vi "Main Tclk.vi"() -> ()   [LabVIEW 2018] (continued)
                        n6809 = Build Path(base path=w1551, name or relative path=w1554) -> (appended path=w1552:path)
                        n6810 = File/Directory Info(path=w1552) -> (path out=w1557:path, error out=w1555:errorcluster)  [unwired: 1 in, 5 out]
                        n6811 = Unbundle By Name(w1555) -> ("status"=w1556:bool)
                        n6812 = case shown="True" w1556 {
                          tunnel: w1557 -> [_ w1571]
                          frame False {
                          }
                          frame True {
                            n6813 = Create Folder(path (use dialog)=w1571) -> ()  [unwired: 1 in, 4 out]
                          }
                        }
                      }
                      frame #1 {
                        n6814 = call "Read FIB Log Files.vi"("Log file path"=path "C:/Program Files (x86)/FEI Company/BDS/LogHVData.log") -> ("HV Data Output"=w1578:T113)  [unwired: 9 in, 1 out]
                        n6815 = Unbundle By Name(w1578) -> ("Filament (A)"=w1594:sgl, "Acclerator (V)"=w1593:sgl, "AccI (uA)"=w1592:sgl, "Extractor (V)"=w1591:sgl, "Emission (uA)"=w1579:sgl, "Suppressor (V)"=w1580:sgl, "SuppI (uA)"=w1590:sgl, "Lens1 (V)"=w1589:sgl, "Lens1I (uA)"=w1588:sgl, "Lens2 (V)"=w1587:sgl, "Lens2I (uA)"=w1586:sgl, "Tip Lifetime (hr)"=w1577:sgl)
                        n6816 = local read "Faraday Cup RT"() -> (w1575:sgl)
                        n6817 = local read "Specimen RT"() -> (w1574:sgl)
                        n6818 = local read "BD1 RT"() -> (w1573:sgl)
                        n6819 = local read "BD2 RT"() -> (w1572:sgl)
                        n6820 = Build Array(w1594, w1593, w1592, w1591, w1579, w1580, w1590, w1589, w1588, w1587, w1586, w1577, w1575, w1574, w1573, w1572) -> (w1582:sgl[])
                        n6821 = Bundle("Suppressor (V)"=w1580, "Emission (uA)"=w1579) -> (w1581:T117)  [unwired: 1 in]
                        n6822 = Add Array Elements(numeric array=w1582) -> (sum=w1583:sgl)
                        n6823 = Equal To 0?(x=w1583) -> (x = 0?=w1585:bool)
                        n6824 = Equal To 0?(x=w1577) -> (x = 0?=w1584:bool)
                        n6825 = And(x=w1585, y=w1584) -> (x .and. y?=w1576:bool)
                        "Re-read HVDataLog" <- w1576
                        n6826 = case shown="False" w1576 {
                          tunnel: w1582 -> [w1599 _]
                          tunnel: w1581 -> [w1603 _]
                          tunnel: w1578 -> [w1596 _]
                          frame False {
                            n6827 = local read "FIB HV DataLog Files"() -> (w1601:path)
                            n6828 = Get Date/Time In Seconds() -> (seconds since 1Jan1904=w1600:timestamp)
                            n6829 = for {
                              tunnel: w1599 -> [w1605] mode=indexing
                              tunnel: [w1604] -> w1598 mode=indexing
                              n6830 = Format Into String(w1605) -> (resulting string=w1604:string)  [unwired: 3 in, 1 out]
                            }
                            n6831 = call "YMD log files.vi"("Input text array"=w1598, "Input header array"=string[] ["Date", "Time", "Filament Current (A)", "Accelerator (V)", "Accelerator I (uA)", "Extractor (V)", "Emission (uA)", "Suppressor (V)", "Suppressor I (uA)", "Lens 1 (V)", "Lens 1 I (uA)", "Lens 2 (V)", "Lens 2 I (uA)", "Tip Lifetime (hr)", "Faraday Cup (nA)", "Specimen (nA)", "Beam Dump 1 (nA)", "Beam Dump 2 (nA)"], "current time"=w1600, "Log file name"="HVDataLog" ("string"), "Log file path"=w1601) -> ()  [unwired: 7 in]
                            "FIB HV DataLog" <- w1603
                            "HV Data Output" <- w1596
                          }
                          frame True {
                          }
                        }
                      }
                    }
                  }
                }
                n6832 = Add(x=w1544, y=w1543) -> (x+y=w1547:u32)
                n6833 = expression code="x*1000"("Interval (s)") -> (w1542:u16)
                n6834 = Less?(x=w1547, y=w1542) -> (x < y?=w1548:bool)
                n6835 = Select(t=w1547, s=w1548, f=u32 0) -> (s? t:f=w1545:u32)
                n6836 = property on="FIB HV DataLog" class="WFChart (strict)"("XScale.Multiplier"="Interval (s)") -> ()  [unwired: 2 in, 2 out]
              }
              frame 1, Default {
              }
              frame 2 {
                n6837 = Equal To 0?(x=w1611) -> (x = 0?=w1614:bool)
                n6838 = local read "Re-read HVDataLog"() -> (w1615:bool)
                n6839 = Or(x=w1614, y=w1615) -> (x .or. y?=w1608:bool)
                n6840 = case shown="True" w1608 {
                  tunnel: w1607 -> [_ w1619]
                  frame False {
                  }
                  frame True {
                    n6841 = stacked-sequence {
                      tunnel: w1619 -> [w1623 _]
                      frame #0 {
                        n6842 = local read "FIB HV DataLog Files"() -> (w1624:path)
                        n6843 = local read "Api"() -> (w1620:refnum<k7>)
                        n6844 = call "SmartSEM Remote API get FIB HV data.vi"("Api in"=w1620) -> ("error out"=w1622:errorcluster, "Capella HV Data Output"=w1621:T17)  [unwired: 7 in, 2 out]
                        n6845 = Get Date/Time In Seconds() -> (seconds since 1Jan1904=w1631:timestamp)
                        n6846 = local write "Capella HV Data Output"(w1621) -> ()
                        n6847 = Format Date/Time String(time format string (%c)="Y%Y\\M%m\\D%d", seconds (now)=w1631) -> (date/time string=w1627:string)  [unwired: 1 out]
                        n6848 = Build Path(base path=w1624, name or relative path=w1627) -> (appended path=w1625:path)
                        n6849 = File/Directory Info(path=w1625) -> (path out=w1630:path, error out=w1628:errorcluster)  [unwired: 1 in, 5 out]
                        n6850 = case shown="True" w1623 {
                          tunnel: w1622 -> [_ _]
                          frame False {
                          }
                          frame True {
                            w1633 = 0.0
                            n6851 = Get Date/Time In Seconds() -> (seconds since 1Jan1904=w1643:timestamp)
                            n6852 = To Double Precision Float(number=w1643) -> (double precision float=w1638:dbl)
                            n6853 = Bundle(w1633, w1633) -> (w1632:cluster{dbl, dbl})  [unwired: 1 in]
                            n6854 = Add(x=w1638, y=86400.0 ("X Scale.Range:Maximum")) -> (x+y=w1640:dbl)
                            n6855 = Initialize Array(w1632, 0) -> (w1635:cluster{dbl, dbl}[])
                            n6856 = Add(x=w1638, y=0.0 ("X Scale.Range:Minimum")) -> (x+y=w1636:dbl)
                            n6857 = property on="FIB HV DataLog" class="WFChart (strict)"("History Data"=w1635, "XScale.Offset"=w1638, "XScale.Minimum"=w1636, "XScale.Maximum"=w1640, "XScale.Increment"=14400.0 ("X Scale.Range:Increment"), "XScale.MinorInc"=3600.0 ("X Scale.Range:Minor Increment")) -> ()  [unwired: 2 in, 2 out]
                          }
                        }
                        n6858 = Unbundle By Name(w1628) -> ("status"=w1629:bool)
                        n6859 = case shown="True" w1629 {
                          tunnel: w1630 -> [_ w1644]
                          frame False {
                          }
                          frame True {
                            n6860 = Create Folder(path (use dialog)=w1644) -> ()  [unwired: 1 in, 4 out]
                          }
                        }
                      }
                      frame #1 {
                        n6861 = local read "Capella HV Data Output"() -> (w1645:T17)
                        n6862 = Unbundle By Name(w1645) -> ("Filament (A)"=w1666:sgl, "Accelerator Target (V)"=w1665:sgl, "Accelerator Actual (V)"=w1664:sgl, "Extrator Target (V)"=w1663:sgl, "Extrator Actual (V)"=w1662:sgl, "Emission Target (uA)"=w1661:sgl, "Emission Actual (uA)"=w1654:sgl, "Suppressor (V)"=w1655:sgl, "Lens1 Target (V)"=w1660:sgl, "Lens1 Actual (V)"=w1659:sgl, "Lens2 Target (V)"=w1658:sgl, "Lens2 Actual (V)"=w1657:sgl, "Tip Lifetime (uAhr)"=w1653:sgl, "Gun Vac (Torr)"=w1652:sgl, "Column Vac (Torr)"=w1651:sgl)
                        n6863 = Bundle("Suppressor (V)"=w1655, "Emission Actual (uA)"=w1654) -> (w1667:T118)  [unwired: 1 in]
                        n6864 = Build Array(w1666, w1665, w1664, w1663, w1662, w1661, w1654, w1655, w1660, w1659, w1658, w1657, w1653) -> (w1656:sgl[])
                        n6865 = Build Array(w1652, w1651) -> (w1650:sgl[])
                        n6866 = local write "FIB HV DataLog"(w1667) -> ()
                        n6867 = for {
                          tunnel: w1656 -> [w1676] mode=indexing
                          tunnel: [w1675] -> w1648 mode=indexing
                          n6868 = Format Into String(w1676) -> (resulting string=w1675:string)  [unwired: 3 in, 1 out]
                        }
                        n6869 = for {
                          tunnel: w1650 -> [w1674] mode=indexing
                          tunnel: [w1673] -> w1647 mode=indexing
                          tunnel: "%e" ("format string") -> [w1672]
                          n6870 = Format Into String(format string=w1672, w1674) -> (resulting string=w1673:string)  [unwired: 2 in, 1 out]
                        }
                        n6871 = Build Array (concatenate)(w1648, w1647) -> (w1646:string[])
                        n6872 = local read "FIB HV DataLog Files"() -> (w1670:path)
                        n6873 = Get Date/Time In Seconds() -> (seconds since 1Jan1904=w1669:timestamp)
                        n6874 = call "YMD log files.vi"("Input text array"=w1646, "Input header array"=string[] ["Date", "Time", "Filament Current (A)", "Accelerator Target (V)", "Accelerator Actual (V)", "Extractor Target (V)", "Extractor Actual (V)", "Emission Target (uA)", "Emission Actual (uA)", "Suppressor (V)", "Lens 1 Target (V)", "Lens 1 Actual (V)", "Lens 2 Target (V)", "Lens 2 Actual (uA)", "Tip Lifetime (hr)", "Gun Vacuum (Torr)", "Column Vacuum (Torr)", ""], "current time"=w1669, "Log file name"="HVDataLog" ("string"), "Log file path"=w1670) -> ()  [unwired: 7 in]
                      }
                    }
                  }
                }
                n6875 = local read "Interval (s)"() -> (w1610:u16)
                n6876 = Add(x=w1612, y=w1611) -> (x+y=w1609:u32)
                n6877 = expression code="x*1000"(w1610) -> (w1616:u16)
                n6878 = Less?(x=w1609, y=w1616) -> (x < y?=w1618:bool)
                n6879 = Select(t=w1609, s=w1618, f=u32 0) -> (s? t:f=w1613:u32)
                n6880 = property on="FIB HV DataLog" class="WFChart (strict)"("XScale.Multiplier"=w1610) -> ()  [unwired: 2 in, 2 out]
              }
            }
          }
        }
        n6881 = case shown="2" w1427 {
          frame 0, Default {
          }
          frame 2 {
            n6882 = local read "Status message"() -> (w1492:string)
            n6883 = Equal?(x=w1492, y="SEM between FIB" ("Status message")) -> (x = y?=w1490:bool)
            n6884 = case shown="False" w1490 {
              frame False {
                n6885 = local read "Api"() -> (w1495:refnum<k7>)
                n6886 = call "SmartSEM Remote API FIB gun state.vi"("Api"=w1495) -> ("error out"=w1493:errorcluster, "FIB Gun State"=w1499:string)  [unwired: 8 in, 1 out]
                "FIB Gun State" <- w1499
                n6887 = case shown="\"Regulating\"" w1499 {
                  tunnel: w1495 -> [_ _ _ _ _ _ _ _ _ _ _ _ _ _ w1522 _ _ _ _ _ _]
                  tunnel: w1493 -> [_ _ _ _ _ _ _ _ _ _ _ _ _ _ w1518 _ _ _ _ _ _]
                  frame "Off", Default {
                    n6888 = property on="Turn off FIB gun" class="Bool (strict)"("DisabledEnum"=T44."Disabled and Grayed Out" ("Disabled")) -> ()  [unwired: 2 in, 2 out]
                    n6889 = property on="Turn on FIB gun" class="Bool (strict)"("DisabledEnum"=T44."Enabled" ("Disabled")) -> ()  [unwired: 2 in, 2 out]
                    n6890 = local write "Turn off FIB gun"(TRUE ("Turn on FIB gun")) -> ()
                    n6891 = local write "Turn on FIB gun"(FALSE ("Turn on FIB gun")) -> ()
                  }
                  frame "On" {
                    w1506 = FALSE ("Turn on FIB gun")
                    w1507 = T44."Enabled" ("Disabled")
                    n6892 = property on="Turn on FIB gun" class="Bool (strict)"("DisabledEnum"=T44."Disabled and Grayed Out" ("Disabled")) -> ()  [unwired: 2 in, 2 out]
                    n6893 = property on="Turn off FIB gun" class="Bool (strict)"("DisabledEnum"=w1507) -> ()  [unwired: 2 in, 2 out]
                    n6894 = property on="Turn FIB gun standby" class="Bool (strict)"("DisabledEnum"=w1507) -> ()  [unwired: 2 in, 2 out]
                    n6895 = local write "Turn on FIB gun"(TRUE ("Turn on FIB gun")) -> ()
                    n6896 = local write "Turn FIB gun standby"(w1506) -> ()
                    n6897 = local write "Turn off FIB gun"(w1506) -> ()
                  }
                  frame "Ramping" {
                  }
                  frame "Error" {
                  }
                  frame "Vac Not Ready" {
                  }
                  frame "Extractor Auto" {
                  }
                  frame "Heating" {
                  }
                  frame "Conditioning" {
                  }
                  frame "Filament Heating" {
                  }
                  frame "Gun colling down" {
                  }
                  frame "Ramping Down" {
                  }
                  frame "Standby" {
                    w1511 = FALSE ("Turn on FIB gun")
                    w1510 = T44."Enabled" ("Disabled")
                    n6898 = property on="Turn on FIB gun" class="Bool (strict)"("DisabledEnum"=w1510) -> ()  [unwired: 2 in, 2 out]
                    n6899 = property on="Turn off FIB gun" class="Bool (strict)"("DisabledEnum"=w1510) -> ()  [unwired: 2 in, 2 out]
                    n6900 = property on="Turn FIB gun standby" class="Bool (strict)"("DisabledEnum"=T44."Disabled and Grayed Out" ("Disabled")) -> ()  [unwired: 2 in, 2 out]
                    n6901 = local write "Turn on FIB gun"(w1511) -> ()
                    n6902 = local write "Turn off FIB gun"(w1511) -> ()
                    n6903 = local write "Turn FIB gun standby"(TRUE ("Turn on FIB gun")) -> ()
                  }
                  frame "FIB Emission Failed" {
                    n6904 = property on="Turn off FIB gun" class="Bool (strict)"("DisabledEnum"=T44."Enabled" ("Disabled")) -> ()  [unwired: 2 in, 2 out]
                    n6905 = property on="Turn on FIB gun" class="Bool (strict)"("DisabledEnum"=T44."Enabled" ("Disabled")) -> ()  [unwired: 2 in, 2 out]
                    n6906 = local write "Turn on FIB gun"(FALSE ("Turn on FIB gun")) -> ()
                    n6907 = local write "Turn off FIB gun"(FALSE ("Turn on FIB gun")) -> ()
                  }
                  frame "Going to regulating" {
                  }
                  frame "Regulating" {
                    w1519 = TRUE ("Turn on FIB gun")
                    w1525 = FALSE ("Turn on FIB gun")
                    w1526 = T44."Enabled" ("Disabled")
                    n6908 = call "SmartSEM Remote API get FIB HV data.vi"("error in"=w1518, "Api in"=w1522) -> ("Capella HV Data Output"=w1520:T17)  [unwired: 6 in, 3 out]
                    "Capella HV Data Output" <- w1520
                    n6909 = property on="Turn on FIB gun" class="Bool (strict)"("DisabledEnum"=T44."Disabled and Grayed Out" ("Disabled")) -> ()  [unwired: 2 in, 2 out]
                    n6910 = property on="Turn off FIB gun" class="Bool (strict)"("DisabledEnum"=w1526) -> ()  [unwired: 2 in, 2 out]
                    n6911 = property on="Turn FIB gun standby" class="Bool (strict)"("DisabledEnum"=w1526) -> ()  [unwired: 2 in, 2 out]
                    n6912 = call "FIB HV target match.vi"("Capella HV Data Output"=w1520) -> ("Max absolute error (V)"=w1523:sgl)  [unwired: 5 in, 5 out]
                    n6913 = Less?(x=w1523, y=sgl 80.0) -> (x < y?=→"FIB HV target matched":bool)
                    n6914 = local write "Turn on FIB gun"(w1519) -> ()
                    n6915 = local write "Start FIB HV DataLog"(w1519) -> ()
                    n6916 = local write "Turn off FIB gun"(w1525) -> ()
                    n6917 = local write "Turn FIB gun standby"(w1525) -> ()
                  }
                  frame "Going to Standby" {
                  }
                  frame "Multi-Heating (Heater is ON)" {
                  }
                  frame "Emission Recovery (Heater is OFF)" {
                  }
                  frame "No User Has Logged On" {
                    n6918 = local write "Status message"("No user has logged on to SmartSEM" ("Status message")) -> ()
                  }
                  frame "No user is logged on" {
                    n6919 = local write "Status message"("No user is logged on to SmartSEM" ("Status message")) -> ()
                  }
                  frame "API not initialized" {
                    n6920 = local write "Status message"("API not initialized" ("Status message")) -> ()
                  }
                }
                n6921 = call "SmartSEM Remote API get string.vi"("error in"=w1493, "lpszParam"="DP_FIB_GUN_VALVE", "Api"=w1495) -> ("data"=w1494:string)  [unwired: 6 in, 2 out]
                n6922 = Concatenate Strings("FIB Gun Valve is " ("lpszCommand"), w1494) -> (→"FIB Gun Valve Status":string)
                n6923 = case shown="\"Closed\", Default" w1494 {
                  frame "Open" {
                    n6924 = local write "Open FIB gun valve"(TRUE ("Open FIB gun valve")) -> ()
                  }
                  frame "Closed", Default {
                    n6925 = local write "Open FIB gun valve"(FALSE ("Open FIB gun valve")) -> ()
                  }
                }
              }
              frame True {
              }
            }
          }
        }
        n6926 = case shown="True" w1428 {
          tunnel: w1427 -> [_ w1486]
          frame False {
          }
          frame True {
            n6927 = case shown="2" w1486 {
              frame 0, Default {
              }
              frame 2 {
                n6928 = local read "Api"() -> (w1489:refnum<k7>)
                n6929 = local read "SEM HV DataLog Files"() -> (w1488:path)
                n6930 = call "SEM HV log.vi"("SEM HV DataLog Files Directory"=w1488, "Api in"=w1489) -> ("SEM HV Data Output"=→"SEM HV Data Output":T16)  [unwired: 7 in, 2 out]
              }
            }
          }
        }
        n6931 = case shown="True" w1415 {
          frame False {
          }
          frame True {
            n6932 = local read "COM port"() -> (w1482:refnum<visa-resource-name>)
            n6933 = local read "Machine Type"() -> (w1483:u8)
            n6934 = local read "Api"() -> (w1484:refnum<k7>)
            n6935 = local read "Current DataLog Files"() -> (w1485:path)
            n6936 = local read "Parameter Names"() -> (w1481:string[])
            n6937 = call "Data log.vi"("COM port"=w1482, "Parameter Names"=w1481, "Machine Type"=w1483, "DataLog Files Directory"=w1485, "Api in"=w1484) -> ()  [unwired: 5 in, 2 out]
          }
        }
        n6938 = local read "Median cycle time est offset (s)"() -> (w1411:i16)
        n6939 = local read "Cycle time array"() -> (w1414:u32[])
        n6940 = Less?(x=w1402, y=u16 10) -> (x < y?=w1400:bool)
        n6941 = Compound Arithmetic op=AND(w1451, w1450, w1443, w1441, w1426, w1404, w1400) -> (w1449:bool)
        n6942 = Array Size(array=w1414) -> (size(s)=w1413:i32)
        n6943 = case shown="True" w1449 {
          tunnel: [w1677 w1680] -> w1448
          tunnel: w1447 -> [w1677 w1679]
          frame False {
          }
          frame True {
            n6944 = local read "FIB slice #"() -> (w1680:u32)
            n6945 = Equal?(x=w1680, y=w1679) -> (x = y?=w1678:bool)
            "SW error warning active" <- w1678
            n6946 = case shown="True" w1678 {
              frame False {
              }
              frame True {
                n6947 = local read "FIB HW Config"() -> (w1684:T23)
                n6948 = Unbundle By Name(w1684) -> ("Beam blank"=w1683:tag)
                n6949 = local read "Api"() -> (w1681:refnum<k7>)
                n6950 = call "FIB beam blank.vi"("Api"=w1681, "Beam blanked"=TRUE, "lines"=w1683) -> ()  [unwired: 2 in, 1 out]
              }
            }
          }
        }
        n6951 = Greater Or Equal?(x=w1413, y=100) -> (x >= y?=w1397:bool)
        n6952 = Select(t=w1411, s=w1397, f=u32 0) -> (s? t:f=w1408:u32)
        n6953 = local read "Est. cycle time (s)"() -> (w1406:u32)
        n6954 = local read "LM overhead"() -> (w1390:u32)
        n6955 = local read "MM overhead"() -> (w1389:u32)
        n6956 = Compound Arithmetic op=ADD(u32 20 ("value"), w1408, w1406, w1390, w1389) -> (w1409:u32)
        "Timeout threshold (s)" <- w1409
        n6957 = expression code="x*1000"(w1409) -> (w1446:u32)
        n6958 = local read "FIB"() -> (w1387:bool)
        n6959 = Less?(x=w1454, y=w1446) -> (x < y?=w1453:bool)
        n6960 = case shown="True" w1387 {
          frame False {
          }
          frame True {
            n6961 = local read "Api"() -> (w1474:refnum<k7>)
            n6962 = call "SmartSEM Remote API get string.vi"("lpszParam"="DP_FIB_IMAGE_PROBE", "Api"=w1474) -> ("data"=w1472:string, "Api out"=w1470:refnum<k7>)  [unwired: 7 in, 1 out]
            n6963 = local write "FIB Milling Probe"(w1472) -> ()
            n6964 = call "SmartSEM Remote API get float.vi"("lpszParam"="AP_FIB_OBJECTIVE_POTENTIAL", "Api"=w1470) -> ("vValue"=w1471:sgl)  [unwired: 7 in, 2 out]
            n6965 = local write "FIB Milling Objective (V)"(w1471) -> ()
          }
        }
        n6966 = Select(t=w1454, s=w1453, f=u32 0) -> (s? t:f=w1455:u32)
        n6967 = case shown="True" "FIB time lapse" {
          tunnel: [u32 0 w1719] -> w1467
          tunnel: w1466 -> [_ w1714]
          tunnel: w1421 -> [_ w1713]
          frame False {
          }
          frame True {
            n6968 = Equal To 0?(x=w1714) -> (x = 0?=w1715:bool)
            n6969 = case shown="True" w1715 {
              frame False {
              }
              frame True {
                n6970 = stacked-sequence {
                  frame #0 {
                    n6971 = local read "File Information"() -> (w1725:T31)
                    n6972 = Get Date/Time In Seconds() -> (seconds since 1Jan1904=w1722:timestamp)
                    n6973 = Unbundle By Name(w1725) -> ("File path"=w1724:path)
                    n6974 = Format Date/Time String(time format string (%c)="Y%Y\\M%m\\D%d", seconds (now)=w1722) -> (date/time string=w1727:string)  [unwired: 1 out]
                    n6975 = Build Path(base path=w1724, name or relative path=w1727) -> (appended path=w1723:path)
                    n6976 = Format Date/Time String(time format string (%c)="%y-%m-%d_%H%M%S") -> (date/time string=w1730:string)  [unwired: 1 in, 1 out]
                    n6977 = File/Directory Info(path=w1723) -> (path out=w1733:path, error out=w1735:errorcluster)  [unwired: 1 in, 5 out]
                    n6978 = Concatenate Strings("FIB_" ("string"), w1730, ".png" ("string")) -> (w1736:string)
                    n6979 = Unbundle By Name(w1735) -> ("status"=w1734:bool)
                    n6980 = Build Path(base path=w1723, name or relative path=w1736) -> (appended path=→"FIB file name":path)
                    n6981 = case shown="True" w1734 {
                      tunnel: w1733 -> [_ w1737]
                      frame False {
                      }
                      frame True {
                        n6982 = Create Folder(path (use dialog)=w1737) -> ()  [unwired: 1 in, 4 out]
                      }
                    }
                  }
                  frame #1 {
                    n6983 = local read "Api"() -> (w1738:refnum<k7>)
                    n6984 = local read "FIB HW Config"() -> (w1744:T23)
                    n6985 = local read "FIB HW Config"() -> (w1741:T23)
                    n6986 = Unbundle By Name(w1744) -> ("Beam blank"=w1743:tag)
                    n6987 = Unbundle By Name(w1741) -> ("FIB Ext Scan"=w1739:tag)
                    n6988 = call "FIB beam blank.vi"("Api"=w1738, "Beam blanked"=TRUE, "lines"=w1743) -> ()  [unwired: 2 in, 1 out]
                    n6989 = call "FIB ext scan.vi"("Ext on"=TRUE ("data"), "FIB Ext Scan"=w1739) -> ()  [unwired: 9 in, 1 out]
                  }
                  frame #2 {
                    n6990 = local read "Machine Type"() -> (w1745:u8)
                    n6991 = case shown="1" w1745 {
                      frame 0, Default {
                      }
                      frame 1 {
                        w1748 = TRUE ("Close session")
                        n6992 = local read "COM port"() -> (w1750:refnum<visa-resource-name>)
                        n6993 = call "Remcon32 command.vi"("Initialization"=w1748, "SEM command"="edx 1", "COM port in"=w1750) -> ("COM port out"=w1749:refnum<visa-resource-name>)  [unwired: 5 in, 3 out]
                        n6994 = call "FIB mode.vi"("Close session"=w1748, "Iterations"=u32 3, "FIB mode"=T10."FIB", "COM port in"=w1749) -> ()  [unwired: 6 in, 2 out]
                      }
                    }
                  }
                  frame #3 {
                    w1754 = TRUE ("As subVi")
                    n6995 = local read "FIB HW Config"() -> (w1755:T23)
                    n6996 = local read "FIB Options"() -> (w1756:T33)
                    n6997 = local read "FIB Scan Parameters"() -> (w1753:T32)
                    n6998 = call "FIB realtime imaging PXIe-6124.vi"("HW Config"=w1755, "Options"=w1756, "Single scan"=w1754, "Scan Para"=w1753, "As subVi"=w1754) -> ()  [unwired: 4 in, 2 out]
                    n6999 = local write "Status message"("FIB imaging" ("Status message")) -> ()
                    n7000 = local write "Image Tabs"(T37."FIB" ("Image Tabs")) -> ()
                  }
                  frame #4 {
                    n7001 = shared-variable ".\\Zeiss Library.lvlib\\FIB Img"() -> (w1759:i16[][])  [unwired: 1 in, 1 out]
                    n7002 = call "16bit Image Normalization.vi"("Transpose"=FALSE, "Input image"=w1759) -> ("Normalized image"=w1762:u8[][])  [unwired: 5 in, 4 out]
                    n7003 = local read "FIB file name"() -> (w1763:path)
                    n7004 = call <vilib>:"Flatten Pixmap.vi"("colors"=u32[] [16777222, 65793, 131586, 197379, 263172, 328965, 394758, 460551, 526344, 592137, 657930, 723723, 789516, 855309, 921102, 986895, 1052688, 1118481, 1184274, 1250067, 1315860, 1381653, 1447446, 1513239, 1579032, 1644825, 1710618, 1776411, 1842204, 1907997, 1973790, 2039583, 2105376, 2171169, 2236962, 2302755, 2368548, 2434341, 2500134, 2565927, 2631720, 2697513, 2763306, 2829099, 2894892, 2960685, 3026478, 3092271, 3158064, 3223857, 3289650, 3355443, 3421236, 3487029, 3552822, 3618615, 3684408, 3750201, 3815994, 3881787, 3947580, 4013373, 4079166, 4144959, 4210752, 4276545, 4342338, 4408131, 4473924, 4539717, 4605510, 4671303, 4737096, 4802889, 4868682, 4934475, 5000268, 5066061, 5131854, 5197647, 5263440, 5329233, 5395026, 5460819, 5526612, 5592405, 5658198, 5723991, 5789784, 5855577, 5921370, 5987163, 6052956, 6118749, 6184542, 6250335, 6316128, 6381921, 6447714, 6513507, 6579300, 6645093, 6710886, 6776679, 6842472, 6908265, 6974058, 7039851, 7105644, 7171437, 7237230, 7303023, 7368816, 7434609, 7500402, 7566195, 7631988, 7697781, 7763574, 7829367, 7895160, 7960953, 8026746, 8092539, 8158332, 8224125, 8289918, 8355711, 8421504, 8487297, 8553090, 8618883, 8684676, 8750469, 8816262, 8882055, 8947848, 9013641, 9079434, 9145227, 9211020, 9276813, 9342606, 9408399, 9474192, 9539985, 9605778, 9671571, 9737364, 9803157, 9868950, 9934743, 10000536, 10066329, 10132122, 10197915, 10263708, 10329501, 10395294, 10461087, 10526880, 10592673, 10658466, 10724259, 10790052, 10855845, 10921638, 10987431, 11053224, 11119017, 11184810, 11250603, 11316396, 11382189, 11447982, 11513775, 11579568, 11645361, 11711154, 11776947, 11842740, 11908533, 11974326, 12040119, 12105912, 12171705, 12237498, 12303291, 12369084, 12434877, 12500670, 12566463, 12632256, 12698049, 12763842, 12829635, 12895428, 12961221, 13027014, 13092807, 13158600, 13224393, 13290186, 13355979, 13421772, 13487565, 13553358, 13619151, 13684944, 13750737, 13816530, 13882323, 13948116, 14013909, 14079702, 14145495, 14211288, 14277081, 14342874, 14408667, 14474460, 14540253, 14606046, 14671839, 14737632, 14803425, 14869218, 14935011, 15000804, 15066597, 15132390, 15198183, 15263976, 15329769, 15395562, 15461355, 15527148, 15592941, 15658734, 15724527, 15790320, 15856113, 15921906, 15987699, 16053492, 16119285, 16185078, 16250871, 16316664, 16382457, 16448250, 16514043, 16579836, 16645629, 16711422, 16448250] ("256 gray scale"), "8-bit pixmap"=w1762) -> ("image data"=w1760:T55)  [unwired: 4 in, 5 out]
                    n7005 = call <vilib>:"Write PNG File.vi"("image data"=w1760, "path to PNG file"=w1763) -> ()  [unwired: 1 in, 9 out]
                  }
                  frame #5 {
                    n7006 = local read "FIB time lapse"() -> (w1764:bool)
                    n7007 = case shown="False" w1764 {
                      tunnel: ["FIB imaging paused" ("Status message") "FIB imaging finished" ("Status message")] -> w1765
                      frame True {
                      }
                      frame False {
                      }
                    }
                    n7008 = local write "Status message"(w1765) -> ()
                  }
                }
              }
            }
            n7009 = Add(x=w1713, y=w1714) -> (x+y=w1717:u32)
            n7010 = expression code="x*1000"("FIB time lapse (s)") -> (w1720:u32)
            n7011 = Less?(x=w1717, y=w1720) -> (x < y?=w1716:bool)
            n7012 = Select(t=w1717, s=w1716, f=u32 0) -> (s? t:f=w1719:u32)
          }
        }
        n7013 = Add(x=w1421, y=w1456) -> (x+y=w1461:u32)
        n7014 = local read "Interval (s)"() -> (w1419:u16)
        n7015 = case shown="False" w1397 {
          tunnel: [w1477 w1479] -> w1398
          tunnel: [w1476 w1480] -> w1399
          tunnel: u32 6618880 ("color(black)") -> [w1477 w1480]
          tunnel: u32 16777216 ("color(black)") -> [w1476 w1479]
          tunnel: [w1475 w1478] -> w1391
          frame True {
            n7016 = local read "Median cycle time (s)"() -> (w1475:u32)
          }
          frame False {
            n7017 = local read "Est. cycle time (s)"() -> (w1478:u32)
          }
        }
        n7018 = local read "Milling para"() -> (w1394:T35)
        n7019 = Add(x=w1421, y=w1429) -> (x+y=w1430:u32)
        n7020 = Add(x=w1421, y=w1418) -> (x+y=w1422:u32)
        n7021 = Less?(x=w1461, y=u32 6000) -> (x < y?=w1458:bool)
        n7022 = expression code="x*1000"(w1419) -> (w1420:u16)
        n7023 = Unbundle By Name(w1394) -> ("Z-step (nm)"=w1386:dbl, "Lines auto pause"=w1384:u16)
        n7024 = Less?(x=w1430, y=u32 10000) -> (x < y?=w1433:bool)
        n7025 = Less?(x=w1422, y=w1420) -> (x < y?=w1424:bool)
        n7026 = property on="Median cycle time (s)" class="DigNum (strict)"("Caption.BGColor"=w1398) -> ()  [unwired: 2 in, 2 out]
        n7027 = property on="Est. cycle time (s)" class="DigNum (strict)"("Caption.BGColor"=w1399) -> ()  [unwired: 2 in, 2 out]
        n7028 = expression code="86400/x"(w1391) -> (w1393:u32)
        n7029 = expression code="x/1000"(w1386) -> (w1385:dbl)
        n7030 = Select(t=w1461, s=w1458, f=u32 0) -> (s? t:f=w1457:u32)
        n7031 = Compound Arithmetic op=MULTIPLY(w1393, w1385, w1384) -> (→"Daily Z removal (um)":dbl)
        n7032 = Select(t=w1430, s=w1433, f=u32 0) -> (s? t:f=w1434:u32)
        n7033 = Select(t=w1422, s=w1424, f=u32 0) -> (s? t:f=w1425:u32)
        n7034 = local read "Stop"() -> (w1464:bool)
      }
      n7035 = while {
        stop <- w1049 stop-if-true
        n7036 = Wait Until Next ms Multiple(millisecond multiple=u32 100) -> ()  [unwired: 1 out]
        n7037 = local read "SEM Options"() -> (w1047:T27)
        n7038 = Unbundle By Name(w1047) -> ("Inverse PNG"=w1046:bool)
        n7039 = stacked-sequence {
          tunnel: w1046 -> [_ _ w1105 _]
          frame #0 {
            n7040 = while {
              stop <- w1067 stop-if-true
              n7041 = local read "3D FIB-SEM Files"() -> (w1063:path)
              n7042 = local read "SEM Scan Parameters"() -> (w1057:T26)
              n7043 = Unbundle By Name(w1057) -> ("Y tiles"=w1058:u8, "X tiles"=w1059:u8)
              n7044 = Wait Until Next ms Multiple(millisecond multiple=u32 100) -> ()  [unwired: 1 out]
              n7045 = Decrement(x=w1058) -> (x-1=w1052:u8)
              n7046 = Decrement(x=w1059) -> (x-1=w1051:u8)
              n7047 = Format Into String(w1052) -> (resulting string=w1056:string)  [unwired: 3 in, 1 out]
              n7048 = Format Into String(w1051) -> (resulting string=w1053:string)  [unwired: 3 in, 1 out]
              n7049 = Concatenate Strings("post_" ("name or relative path"), w1056, "-" ("name or relative path"), w1053, ".png" ("name or relative path")) -> (w1055:string)
              n7050 = Build Path(base path=w1063, name or relative path=w1055) -> (appended path=w1064:path)
              n7051 = File/Directory Info(path=w1064) -> (error out=w1065:errorcluster)  [unwired: 1 in, 6 out]
              n7052 = Unbundle By Name(w1065) -> ("status"=w1062:bool)
              n7053 = local read "Stop"() -> (w1066:bool)
              n7054 = Not(x=w1062) -> (.not. x?=w1061:bool)
              n7055 = Or(x=w1061, y=w1066) -> (x .or. y?=w1067:bool)
            }
          }
          frame #1 {
            n7056 = local read "3D FIB-SEM Files"() -> (w1071:path)
            n7057 = local read "SEM Scan Parameters"() -> (w1079:T26)
            n7058 = Unbundle By Name(w1079) -> ("Y tiles"=w1070:u8, "X tiles"=w1069:u8)
            n7059 = Decrement(x=w1070) -> (x-1=w1075:u8)
            n7060 = Decrement(x=w1069) -> (x-1=w1074:u8)
            n7061 = Format Into String(w1075) -> (resulting string=w1078:string)  [unwired: 3 in, 1 out]
            n7062 = Format Into String(w1074) -> (resulting string=w1076:string)  [unwired: 3 in, 1 out]
            n7063 = Concatenate Strings("pre_" ("name or relative path"), w1078, "-" ("name or relative path"), w1076, ".png" ("name or relative path")) -> (w1073:string)
            n7064 = Build Path(base path=w1071, name or relative path=w1073) -> (appended path=w1083:path)
            n7065 = File/Directory Info(path=w1083) -> (error out=w1082:errorcluster)  [unwired: 1 in, 6 out]
            n7066 = Unbundle By Name(w1082) -> ("status"=w1072:bool)
            n7067 = case shown="True" w1072 {
              tunnel: w1071 -> [_ w1086]
              tunnel: w1070 -> [_ w1085]
              tunnel: w1069 -> [_ w1084]
              frame False {
              }
              frame True {
                n7068 = for {
                  N: w1085 -> [_]
                  tunnel: w1086 -> [w1088]
                  tunnel: w1084 -> [w1087]
                  i -> [w1089]
                  n7069 = for {
                    N: w1087 -> [_]
                    tunnel: w1089 -> [w1099]
                    tunnel: w1088 -> [w1090]
                    i -> [w1100]
                    n7070 = Format Into String(w1099) -> (resulting string=w1102:string)  [unwired: 3 in, 1 out]
                    n7071 = Format Into String(w1100) -> (resulting string=w1104:string)  [unwired: 3 in, 1 out]
                    n7072 = Concatenate Strings(w1102, "-" ("name or relative path"), w1104, ".png" ("name or relative path")) -> (w1091:string)
                    n7073 = Concatenate Strings("post_" ("name or relative path"), w1091) -> (w1095:string)
                    n7074 = Concatenate Strings("pre_" ("name or relative path"), w1091) -> (w1096:string)
                    n7075 = Build Path(base path=w1090, name or relative path=w1095) -> (appended path=w1092:path)
                    n7076 = Build Path(base path=w1090, name or relative path=w1096) -> (appended path=w1093:path)
                    n7077 = Move(source path=w1092, 9:TRUE ("overwrite (F)"), 10:w1093) -> ()  [unwired: 2 in, 3 out]
                  }
                }
              }
            }
          }
          frame #2 {
            n7078 = local read "3D FIB-SEM Files"() -> (w1108:path)
            n7079 = local read "SEM Scan Parameters"() -> (w1116:T26)
            n7080 = Unbundle By Name(w1116) -> ("Y tiles"=w1107:u8, "X tiles"=w1106:u8)
            n7081 = Decrement(x=w1107) -> (x-1=w1112:u8)
            n7082 = Decrement(x=w1106) -> (x-1=w1111:u8)
            n7083 = Format Into String(w1112) -> (resulting string=w1115:string)  [unwired: 3 in, 1 out]
            n7084 = Format Into String(w1111) -> (resulting string=w1113:string)  [unwired: 3 in, 1 out]
            n7085 = Concatenate Strings("post_" ("name or relative path"), w1115, "-" ("name or relative path"), w1113, ".png" ("name or relative path")) -> (w1110:string)
            n7086 = Build Path(base path=w1108, name or relative path=w1110) -> (appended path=w1120:path)
            n7087 = File/Directory Info(path=w1120) -> (error out=w1119:errorcluster)  [unwired: 1 in, 6 out]
            n7088 = Unbundle By Name(w1119) -> ("status"=w1109:bool)
            n7089 = case shown="False" w1109 {
              tunnel: w1108 -> [w1144 _]
              tunnel: w1107 -> [w1143 _]
              tunnel: w1106 -> [w1142 _]
              tunnel: w1105 -> [w1128 _]
              frame False {
                n7090 = for {
                  N: w1143 -> [_]
                  tunnel: w1144 -> [w1151]
                  tunnel: w1142 -> [w1150]
                  tunnel: [w1149] -> w1132 mode=indexing
                  tunnel: [w1148] -> w1131 mode=indexing
                  tunnel: [w1147] -> w1130 mode=indexing
                  tunnel: w1128 -> [w1146]
                  tunnel: [w1145] -> w1127 mode=indexing
                  i -> [w1152]
                  n7091 = for {
                    N: w1150 -> [_]
                    tunnel: w1152 -> [w1169]
                    tunnel: w1151 -> [w1168]
                    tunnel: [w1155] -> w1149 mode=indexing
                    tunnel: [w1156] -> w1148 mode=indexing
                    tunnel: [w1157] -> w1147 mode=indexing
                    tunnel: w1146 -> [w1167]
                    tunnel: [w1166] -> w1145 mode=indexing
                    i -> [w1170]
                    n7092 = Format Into String(w1169) -> (resulting string=w1163:string)  [unwired: 3 in, 1 out]
                    n7093 = Format Into String(w1170) -> (resulting string=w1165:string)  [unwired: 3 in, 1 out]
                    n7094 = Concatenate Strings(w1163, "-" ("name or relative path"), w1165, ".png" ("name or relative path")) -> (w1161:string)
                    n7095 = Concatenate Strings("post_" ("name or relative path"), w1161) -> (w1159:string)
                    n7096 = Concatenate Strings("pre_" ("name or relative path"), w1161) -> (w1158:string)
                    n7097 = call "SIFT align.vi"("post image file"=w1158, "pre image file"=w1159, "Inverse PNG"=w1167, "Affine"=FALSE, "working directory"=w1168) -> ("Delta image"=w1155:dbl, "failed"=w1166:bool, "Delta Y"=w1156:dbl, "Delta X"=w1157:dbl)  [unwired: 3 in]
                  }
                }
                "Align failed array" <- w1127
                n7098 = local read "SEM Scan Parameters"() -> (w1126:T26)
                n7099 = Array Size(array=w1132) -> (size(s)=w1133:i32[])
                n7100 = Array Size(array=w1131) -> (size(s)=w1138:i32[])
                n7101 = Array Size(array=w1130) -> (size(s)=w1139:i32[])
                n7102 = Multiply Array Elements(1:w1133) -> (0:w1134:i32)
                n7103 = Multiply Array Elements(1:w1138) -> (0:w1137:i32)
                n7104 = Multiply Array Elements(1:w1139) -> (0:w1140:i32)
                n7105 = Reshape Array(w1132, w1134) -> (w1135:dbl[])
                n7106 = Reshape Array(w1131, w1137) -> (w1136:dbl[])
                n7107 = Reshape Array(w1130, w1140) -> (w1141:dbl[])
                n7108 = call-poly <vilib>:"Mean.vi"("X"=w1135) -> ("mean"=→"Delta image":dbl)  [unwired: 1 out]
                n7109 = call-poly <vilib>:"Mean.vi"("X"=w1136) -> ("mean"=w1123:dbl)  [unwired: 1 out]
                n7110 = Unbundle By Name(w1126) -> ("Pixel size (nm)"=w1121:sgl)
                n7111 = call-poly <vilib>:"Mean.vi"("X"=w1141) -> ("mean"=w1125:dbl)  [unwired: 1 out]
                n7112 = Multiply(x=w1123, y=w1121) -> (x*y=→"Delta Y":dbl)
                n7113 = Multiply(x=w1125, y=w1121) -> (x*y=→"Delta X":dbl)
              }
              frame True {
              }
            }
          }
          frame #3 {
            n7114 = local read "3D FIB-SEM Files"() -> (w1173:path)
            n7115 = local read "SEM Scan Parameters"() -> (w1181:T26)
            n7116 = Unbundle By Name(w1181) -> ("Y tiles"=w1172:u8, "X tiles"=w1171:u8)
            n7117 = Decrement(x=w1172) -> (x-1=w1177:u8)
            n7118 = Decrement(x=w1171) -> (x-1=w1176:u8)
            n7119 = Format Into String(w1177) -> (resulting string=w1180:string)  [unwired: 3 in, 1 out]
            n7120 = Format Into String(w1176) -> (resulting string=w1178:string)  [unwired: 3 in, 1 out]
            n7121 = Concatenate Strings("post_" ("name or relative path"), w1180, "-" ("name or relative path"), w1178, ".png" ("name or relative path")) -> (w1175:string)
            n7122 = Build Path(base path=w1173, name or relative path=w1175) -> (appended path=w1185:path)
            n7123 = File/Directory Info(path=w1185) -> (error out=w1184:errorcluster)  [unwired: 1 in, 6 out]
            n7124 = Unbundle By Name(w1184) -> ("status"=w1174:bool)
            n7125 = case shown="False" w1174 {
              tunnel: w1173 -> [w1188 _]
              tunnel: w1172 -> [w1187 _]
              tunnel: w1171 -> [w1186 _]
              frame False {
                n7126 = for {
                  N: w1187 -> [_]
                  tunnel: w1188 -> [w1190]
                  tunnel: w1186 -> [w1189]
                  i -> [w1191]
                  n7127 = for {
                    N: w1189 -> [_]
                    tunnel: w1191 -> [w1201]
                    tunnel: w1190 -> [w1193]
                    i -> [w1202]
                    n7128 = Format Into String(w1201) -> (resulting string=w1204:string)  [unwired: 3 in, 1 out]
                    n7129 = Format Into String(w1202) -> (resulting string=w1206:string)  [unwired: 3 in, 1 out]
                    n7130 = Concatenate Strings(w1204, "-" ("name or relative path"), w1206, ".png" ("name or relative path")) -> (w1192:string)
                    n7131 = Concatenate Strings("post_" ("name or relative path"), w1192) -> (w1197:string)
                    n7132 = Concatenate Strings("pre_" ("name or relative path"), w1192) -> (w1198:string)
                    n7133 = Build Path(base path=w1193, name or relative path=w1197) -> (appended path=w1194:path)
                    n7134 = Build Path(base path=w1193, name or relative path=w1198) -> (appended path=w1195:path)
                    n7135 = Move(source path=w1194, 9:TRUE ("overwrite (F)"), 10:w1195) -> ()  [unwired: 2 in, 3 out]
                  }
                }
              }
              frame True {
              }
            }
          }
        }
        n7136 = local read "Stop"() -> (w1049:bool)
      }
    }
    frame #4 {
      w9445 = sgl[] [] ("FI array")
      w9435 = T44."Enabled" ("Disabled")
      w9447 = FALSE ("Off")
      n7137 = local read "Hardware Configuration"() -> (w9443:T25)
      n7138 = property on="Mill start from Last" class="Bool (strict)"("DisabledEnum"=w9435) -> ()  [unwired: 2 in, 2 out]
      n7139 = local write "Stop"(w9447) -> ()
      n7140 = local write "Off"(w9447) -> ()
      n7141 = local write "3D FIB-SEM"(w9447) -> ()
      n7142 = local write "Scan x1"(w9447) -> ()
      n7143 = local write "Scan xn"(w9447) -> ()
      n7144 = local write "FIB time lapse"(w9447) -> ()
      n7145 = property on="Scan x1" class="Bool (strict)"("DisabledEnum"=w9435) -> ()  [unwired: 2 in, 2 out]
      n7146 = property on="Scan xn" class="Bool (strict)"("DisabledEnum"=w9435) -> ()  [unwired: 2 in, 2 out]
      n7147 = property on="FIB Imaging" class="Bool (strict)"("DisabledEnum"=w9435) -> ()  [unwired: 2 in, 2 out]
      n7148 = property on="FIB time lapse" class="Bool (strict)"("DisabledEnum"=w9435) -> ()  [unwired: 2 in, 2 out]
      n7149 = property on="Reset" class="Bool (strict)"("DisabledEnum"=w9435) -> ()  [unwired: 2 in, 2 out]
      n7150 = property on="Pre image" class="Bool (strict)"("DisabledEnum"=w9435) -> ()  [unwired: 2 in, 2 out]
      n7151 = property on="Post image" class="Bool (strict)"("DisabledEnum"=w9435) -> ()  [unwired: 2 in, 2 out]
      n7152 = shared-variable "My Computer\\Zeiss Library.lvlib\\Stop"(w9447) -> ()  [unwired: 1 in, 1 out]
      n7153 = Unbundle By Name(w9443) -> ("SEM X coil"=w9438:refnum<k15>, "SEM Y coil"=w9437:refnum<k15>, "SEM Detectors"=w9436:refnum<k15>)
      n7154 = property on="FIB Profile" class="Bool (strict)"("DisabledEnum"=w9435) -> ()  [unwired: 2 in, 2 out]
      n7155 = property on="Start Current DataLog" class="Bool (strict)"("DisabledEnum"=w9435) -> ()  [unwired: 2 in, 2 out]
      n7156 = property on="Beam blanked" class="Bool (strict)"("DisabledEnum"=w9435) -> ()  [unwired: 2 in, 2 out]
      n7157 = property on="Spot" class="Bool (strict)"("DisabledEnum"=w9435) -> ()  [unwired: 2 in, 2 out]
      n7158 = property on="ROI" class="Bool (strict)"("DisabledEnum"=w9435) -> ()  [unwired: 2 in, 2 out]
      n7159 = property on="Mill Stop" class="Bool (strict)"("DisabledEnum"=w9435) -> ()  [unwired: 2 in, 2 out]
      n7160 = property on="Mill" class="Bool (strict)"("DisabledEnum"=w9435) -> ()  [unwired: 2 in, 2 out]
      n7161 = property on="FIB FOV (um)" class="DigNum (strict)"("DisabledEnum"=w9435) -> ()  [unwired: 2 in, 2 out]
      n7162 = property on="X resolution" class="DigNum (strict)"("DisabledEnum"=w9435) -> ()  [unwired: 2 in, 2 out]
      n7163 = property on="Z resolution" class="DigNum (strict)"("DisabledEnum"=w9435) -> ()  [unwired: 2 in, 2 out]
      n7164 = property on="Z-step (nm)" class="DigNum (strict)"("DisabledEnum"=w9435) -> ()  [unwired: 2 in, 2 out]
      n7165 = property on="X center (um)" class="DigNum (strict)"("DisabledEnum"=w9435) -> ()  [unwired: 2 in, 2 out]
      n7166 = property on="Z center (um)" class="DigNum (strict)"("DisabledEnum"=w9435) -> ()  [unwired: 2 in, 2 out]
      n7167 = property on="X size (um)" class="DigNum (strict)"("DisabledEnum"=w9435) -> ()  [unwired: 2 in, 2 out]
      n7168 = property on="Z size (um)" class="DigNum (strict)"("DisabledEnum"=w9435) -> ()  [unwired: 2 in, 2 out]
      n7169 = Build Array(w9438, w9437) -> (w9439:refnum<k15>[])
      n7170 = call <instrlib>:"niScope Abort.vi"("instrument handle"=w9436) -> ("instrument handle out"=w9441:refnum<k15>, "error out"=w9440:errorcluster)  [unwired: 13 in]
      n7171 = call <instrlib>:"niScope Close.vi"("instrument handle"=w9441, "error in"=w9440) -> ("error out"=w9442:errorcluster)  [unwired: 13 in]
      n7172 = local read "Machine Type"() -> (w9444:u8)
      n7173 = for {
        tunnel: w9439 -> [w9452] mode=indexing
        shift-right: [w9449] -> _
        shift-left: w9442 -> [w9451]
        n7174 = call <instrlib>:"niFgen Abort Generation.vi"("error in (no error)"=w9451, "Instrument Handle"=w9452) -> ("error out"=w9450:errorcluster, "Instrument Handle Out"=w9448:refnum<k15>)  [unwired: 8 in]
        n7175 = call <instrlib>:"niFgen Close.vi"("error in (no error)"=w9450, "Instrument Handle"=w9448) -> ("error out"=w9449:errorcluster)  [unwired: 9 in]
      }
      n7176 = local write "Delta Z array"(w9445) -> ()
      n7177 = local write "Delta X sum array"(w9445) -> ()
      n7178 = local write "Delta Y sum array"(w9445) -> ()
      n7179 = local write "Delta image array"(w9445) -> ()
      n7180 = local write "Milling Z voltage array"(w9445) -> ()
      n7181 = local write "Re-engage Delta X array"(w9445) -> ()
      n7182 = local write "Re-engage Delta Y array"(w9445) -> ()
      n7183 = local write "Re-engage X shift array"(w9445) -> ()
      n7184 = local write "Re-engage Y shift array"(w9445) -> ()
      n7185 = local write "FI grid array tiled"(sgl[][][][][] [] ("FI grid array tiled")) -> ()
      n7186 = local write "FI array"(w9445) -> ()
      n7187 = local write "Temp array"(w9445) -> ()
